vi "OracleLoop.vi"(8 "Error In":errorcluster, 11 "Message Queues":T1) -> (0 "Error Out":errorcluster)   [LabVIEW 2017, in "Server.lvlib" / "Oracle.lvlib"]
doc: "This Loop is responsible for polling the Oracle Database for new SRs. It will then transfer these SRs to the MHL for further processing.\nThis Loop does not have its own queue. Thats why it is stopped with the \"Stop?\" Global Variable!"
uses:
  Oracle.lvlib
  Message Queue/CommReferences.ctl
  Message Queue/MessageCluster.ctl
  <vilib>/Utility/error.llb/Error Cluster From Error Code.vi
  Message Queue/EnqueueMessage(Single).vi
  <vilib>/ErrorRing/Error Ring.xnode
  Message Queue/Message Queue.lvlib
  ErrorLogger/ErrorLogger.lvlib
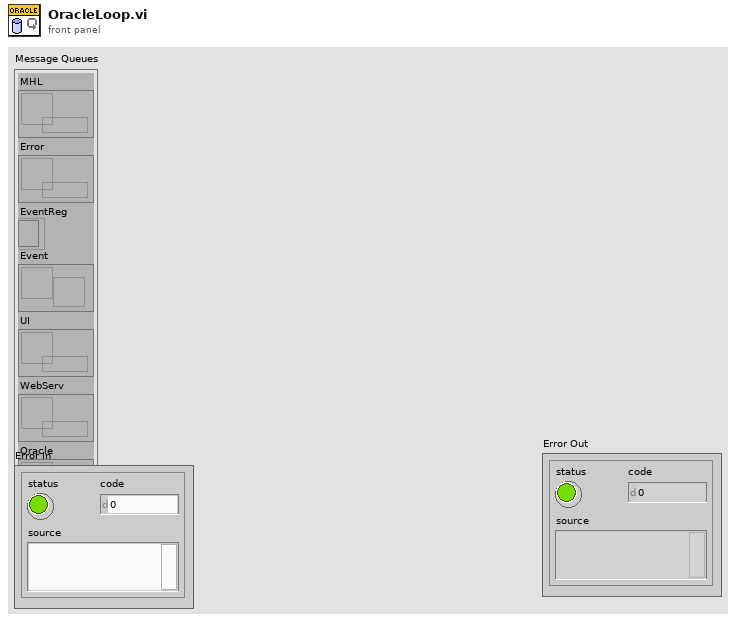
[diagram p1: front panel]
types:
  T1 = typedef "Server.lvlib/Message Queue.lvlib/CommReferences.ctl" = cluster{"MHL":refnum<queue>, "Error":refnum<queue>, "EventReg":refnum<event-registration>, "Event":refnum<user-event>, "UI":refnum<queue>, "WebServ":refnum<queue>, "Oracle":refnum<queue>}
  T2 = typedef "Server.lvlib/SR List.ctl" = T3[]
  T3 = typedef "Server.lvlib/SR Data.ctl" = cluster{"SR#":dbl, "Group":string, "Owner":string, "Problem Summary":string, "Last Updated":timestamp, "Customer First Name":string, "Customer Last Name":string, "Company":string, "Created On":timestamp, "SR Type":string, "Status":string, "Service Level":string, "Channel":string, "Days Open":dbl}
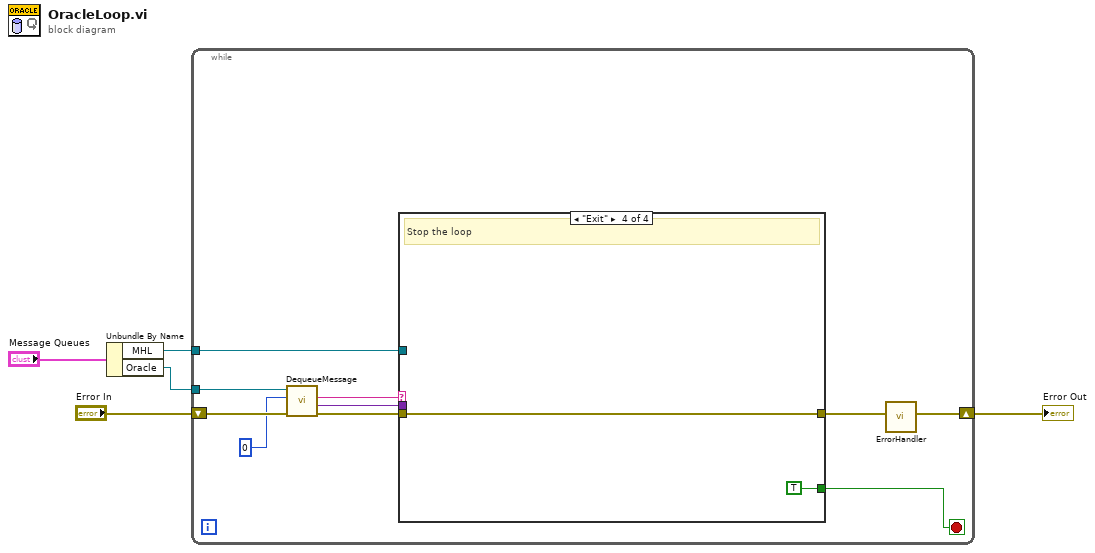
[diagram p0: block diagram]
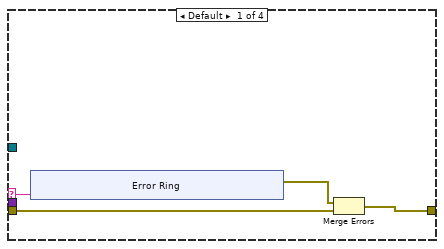
[diagram p2: hidden frame]
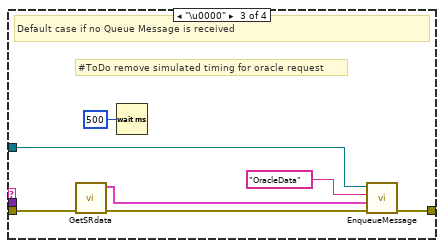
[diagram p4: hidden frame]
diagram:
  n1 = Unbundle By Name("Message Queues") -> ("MHL"=w2:refnum<queue>, "Oracle"=w1:refnum<queue>)
  n2 = while {
    shift-right: [w12] -> w4
    shift-left: "Error In" -> [w15]
    tunnel: w2 -> [w13]
    tunnel: w1 -> [w10]
    stop <- w6 stop-if-true
    n3 = call "DequeueMessage.vi"("error in (no error)"=w15, "timeout ms (-1)"=0, "Message Queue"=w10) -> ("error out"=w11:errorcluster, "Message Data"=w8:variant, "Message"=w9:string)  [unwired: 4 in, 2 out]
    n4 = case shown="\"Exit\"" w9 {
      selector: w9 -> [w18 _ _ _]
      tunnel: w11 -> [w19 w27 w34 w36]
      tunnel: [w17 w27 w33 w36] -> w14
      tunnel: w13 -> [_ _ w32 _]
      tunnel: w8 -> [_ _ _ _]
      tunnel: [_ _ _ TRUE] -> w6
      frame Default {
        n5 = xnode "Error Ring"("parameter 0"=w18) -> ("error out"=w16:errorcluster)
        n6 = Merge Errors(w16, w19) -> (w17:errorcluster)
      }
      frame "Initialize" {
        # "#ToDo Open Oracle Connection here"
      }
      frame "\u0000" {
        # "#ToDo remove simulated timing for oracle request"
        # "Default case if no Queue Message is received"
        n7 = call "GetSRdata.vi"("Error In"=w34) -> ("Error Out"=w30:errorcluster, "SRList"=w29:T2)  [unwired: 9 in]
        n8 = Wait (ms)(milliseconds to wait=u32 500) -> ()  [unwired: 1 out]
        n9 = call-poly "EnqueueMessage.vi"("error in (no error)"=w30, "Message Data"=w29, "Message"="OracleData", "Message Queue"=w32) -> ("error out"=w33:errorcluster)  [unwired: 6 in, 1 out]
      }
      frame "Exit" {
        # "Stop the loop"
      }
    }
    n10 = call "ErrorHandler.vi"("Error In"=w14) -> ("Error Out"=w12:errorcluster)  [unwired: 10 in]
  }
  "Error Out" <- w4
